vi "drawCircle.vi"(8 "error in":errorcluster, 9 "diameter":i32, 10 "center (x,y)":i32[](array[numeric]), 11 "Image in":T1) -> (0 "error out":errorcluster, 3 "Image out":T1)   [LabVIEW 2015]
uses:
  <vilib>/vision/Image Controls.llb/IMAQ Image.ctl
panel:
  in  "line width":i32=5
  # "draw cicle"
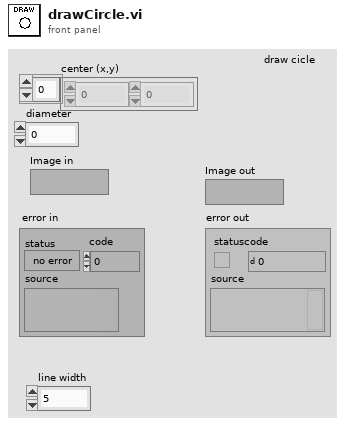
[diagram p1: front panel]
types:
  T1 = typedef "IMAQ Image.ctl" = refnum<image>
  T2 = cluster{"Left":i32, "Top":i32, "Right":i32, "Bottom":i32}
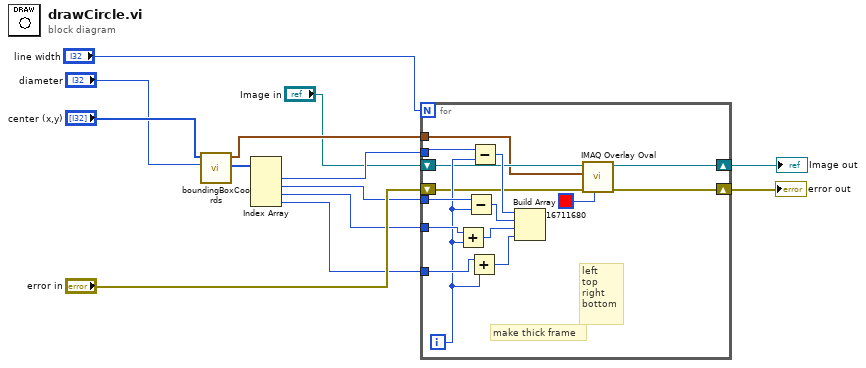
[diagram p0: block diagram]
diagram:
  n1 = call "boundingBoxCoords.vi"("side length (px)"="diameter", "center (x,y)"="center (x,y)") -> ("bounding rectangle"=w7:i32[], "bounding box"=w2:T2)  [unwired: 8 in]
  n2 = Index Array(array=w7) -> (element #1=w6:i32, element #2=w5:i32, element #3=w4:i32, element #4=w3:i32)  [unwired: 4 in]
  n3 = for {
    N: "line width" -> [_]
    tunnel: w5 -> [w26]
    tunnel: w3 -> [w22]
    tunnel: w4 -> [w24]
    tunnel: w6 -> [w28]
    shift-right: [w18] -> w13
    shift-left: "Image in" -> [w19]
    shift-right: [w17] -> w12
    shift-left: "error in" -> [w16]
    tunnel: w2 -> [w15]
    i -> [w21]
    # "make thick frame"
    # "left\ntop\nright\nbottom"
    n4 = Add(x=w24, y=w21) -> (x+y=w23:i32)
    n5 = Subtract(x=w26, y=w21) -> (x-y=w25:i32)
    n6 = Add(x=w22, y=w21) -> (x+y=w20:i32)
    n7 = Subtract(x=w28, y=w21) -> (x-y=w27:i32)
    n8 = Build Array(w27, w25, w23, w20) -> ()  [unwired: 1 out]
    n9 = call "IMAQ Overlay Oval"("Color"=u32 16711680, "error in (no error)"=w16, "Bounding Rectangle"=w15, "Image"=w19) -> ("error out"=w17:errorcluster, "Image Out"=w18:T1)  [unwired: 6 in]
  }
  "Image out" <- w13
  "error out" <- w12
